vi "CRYAuto Listbox Cell Width.vi"(11 "Listbox In":refnum<vi>) -> (3 "Listbox out":refnum<vi>)   [LabVIEW 2013]
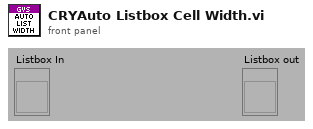
[diagram p1: front panel]
types:
  T1 = cluster{"left":i16, "top":i16, "right":i16, "bottom":i16}
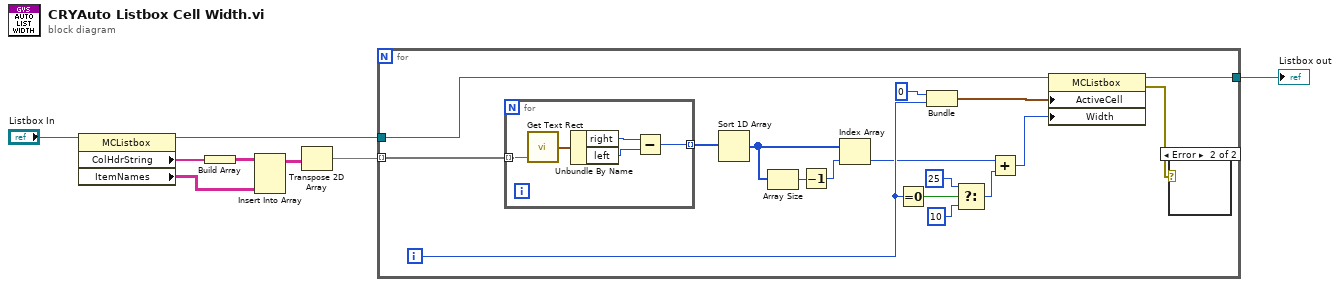
[diagram p0: block diagram]
diagram:
  n1 = property class="MCListbox"(reference="Listbox In") -> (reference out=w6:refnum<vi>, "ColHdrString"=w4:string[], "ItemNames"=w2:string[][])  [unwired: 1 in, 1 out]
  n2 = Build Array(w4) -> (w3:string[][])
  n3 = Insert Into Array(array=w3, new element=w2) -> (w1:string[][])  [unwired: 2 in]
  n4 = Transpose 2D Array(2D array=w1) -> (transposed array=w8:string[][])
  n5 = for {
    tunnel: w8 -> [w25] mode=indexing
    tunnel: w6 -> [w24]
    tunnel: [w23] -> w5
    i -> [w22]
    n6 = for {
      tunnel: w25 -> [w30] mode=indexing
      tunnel: [w26] -> w13 mode=indexing
      n7 = call <vilib>:"Get Text Rect.vi"("text"=w30) -> ("rect"=w29:T1)  [unwired: 5 in, 3 out]
      n8 = Unbundle By Name(w29) -> ("right"=w27:i16, "left"=w28:i16)
      n9 = Subtract(x=w27, y=w28) -> (x-y=w26:i16)
    }
    n10 = Sort 1D Array(array=w13) -> (sorted array=w12:i16[])
    n11 = Array Size(array=w12) -> (size(s)=w11:i32)
    n12 = Decrement(x=w11) -> (x-1=w10:i32)
    n13 = Index Array(array=w12, index=w10) -> (element=w14:i16)
    n14 = Equal To 0?(x=w22) -> (x = 0?=w18:bool)
    n15 = Bundle("Numeric"=i16 0, w22) -> (w20:cluster{"Numeric":i16, i32})  [unwired: 1 out]
    n16 = Select(t=i16 25 ("y"), s=w18, f=i16 10 ("y")) -> (s? t:f=w15:i16)
    n17 = Add(x=w14, y=w15) -> (x+y=w19:i16)
    n18 = property class="MCListbox"(reference=w24, "ActiveCell"=w20, "Width"=w19) -> (reference out=w23:refnum<vi>, error out=w9:errorcluster)  [unwired: 1 in]
    n19 = case shown="Error" w9 {
      frame No Error {
      }
      frame Error {
      }
    }
  }
  "Listbox out" <- w5
